vi "DSP_RegisterRead.vi"(3 "error in (no error)":errorcluster, 4 "Offset":u32, 5 "Board Handle":u64) -> (0 "error out":errorcluster, 1 "Value":u32, 2 "Board Handle Out":u64)   [LabVIEW 2009]
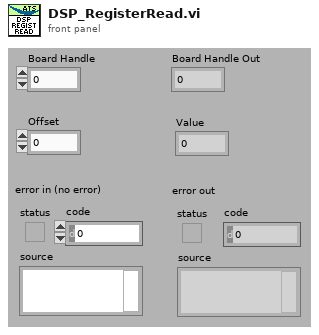
[diagram p1: front panel]
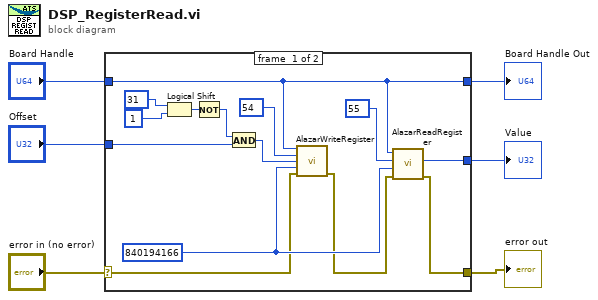
[diagram p0: block diagram]
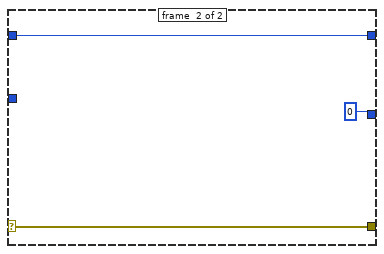
[diagram p2: hidden frame]
diagram:
  n1 = case shown="No Error" "error in (no error)" {
    selector: "error in (no error)" -> [w13 w23]
    tunnel: [w8 w23] -> w5
    tunnel: [w15 w22] -> w4
    tunnel: "Board Handle" -> [w15 w22]
    tunnel: "Offset" -> [w16 _]
    tunnel: [w7 u32 0] -> w1
    frame #0 {
      w14 = u32 840194166
      n2 = Logical Shift(y=31, x=u32 1) -> (x << y=w18:u32)
      n3 = Not(x=w18) -> (.not. x?=w17:u32)
      n4 = And(x=w17, y=w16) -> (x .and. y?=w10:u32)
      n5 = call "AlazarWriteRegister.vi"("Board Handle"=w15, "Offset"=u32 54, "Value"=w10, "Password"=w14, "error in (no error)"=w13) -> ("error out"=w12:errorcluster)  [unwired: 8 in, 2 out]
      n6 = call "AlazarReadRegister.vi"("error in (no error)"=w12, "Password"=w14, "Offset"=u32 55, "Board Handle"=w15) -> ("error out"=w8:errorcluster, "Value Out"=w7:u32)  [unwired: 2 out]
    }
    frame #1 {
    }
  }
  "Board Handle Out" <- w4
  "error out" <- w5
  "Value" <- w1
